vi "Get Installed Software.vi"   [LabVIEW 2014, in "nisyscfg.lvlib"]
doc: "Retrieves the software installed on a system."
uses:
  nisyscfg.lvlib
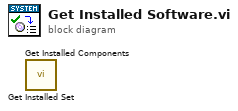
[diagram p0: block diagram]
diagram:
  n1 = call "Get Installed Set.vi"() -> ()  [unwired: 9 in, 3 out]
  n2 = call "Get Installed Components.vi"() -> ()  [unwired: 9 in, 3 out]
